vi "ExWrite8BitTiff.vi"() -> ()   [LabVIEW 2010]
panel:
  in  "File Name":path
  out "error out":errorcluster
  in  "error in (no error)":errorcluster
  in  "X Size":u32=1 min=1 step=1
  in  "Y Size":u32=1 min=1 step=1
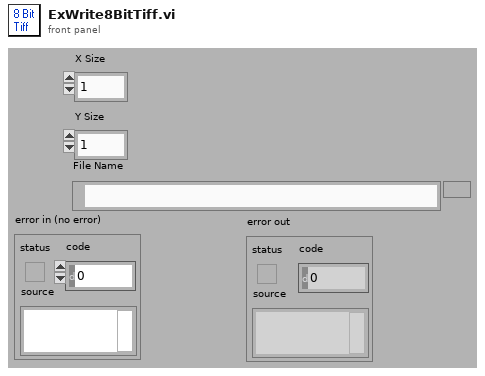
[diagram p1: front panel]
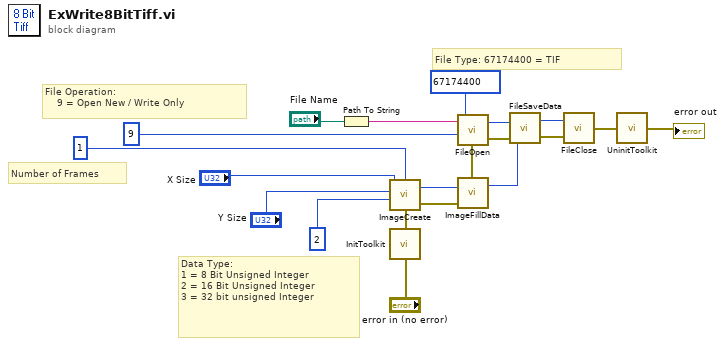
[diagram p0: block diagram]
diagram:
  # "Data Type:\n1 = 8 Bit Unsigned Integer\n2 = 16 Bit Unsigned Integer\n3 = 32 bit unsigned Integer"
  # "File Type: 67174400 = TIF"
  # "Number of Frames"
  # "File Operation:\n    9 = Open New / Write Only"
  n1 = Path To String(path="File Name") -> (string=w1:string)
  n2 = call <userlib>:"InitToolkit.vi"("error in"="error in (no error)") -> ("error out"=w10:errorcluster)
  n3 = call <userlib>:"ImageCreate.vi"("X dimension"="X Size", "Y dimension"="Y Size", "Data Type"=u16 2, "error in"=w10, "Number Of Frames"=1) -> ("Image Handle"=w19:u32, "error out"=w20:errorcluster)
  n4 = call <userlib>:"ImageFillData.vi"("error in"=w20, "Image Handle"=w19) -> ("error out"=w14:errorcluster, "Image Handle"=w17:u32)  [unwired: 1 in]
  n5 = call <userlib>:"FileOpen.vi"("error in"=w14, "File Operations"=9, "FileName"=w1, "File Type"=67174400 ("Numeric")) -> ("error out"=w13:errorcluster, "File Handle"=w12:u32)
  n6 = call <userlib>:"FileSaveData.vi"("error in"=w13, "Image Handle"=w17, "File Handle"=w12) -> ("error out"=w18:errorcluster, "File Handle"=w16:u32)
  n7 = call <userlib>:"FileClose.vi"("error in"=w18, "File Handle"=w16) -> ("error out"=w11:errorcluster)
  n8 = call <userlib>:"UninitToolkit.vi"("error in"=w11) -> ("error out"=→"error out":errorcluster)
